vi "Write Configuration.vi"(8 "error in (no error)":errorcluster, 10 "Configuration.lvlibp:Configuration.lvclass":refnum<class "Configuration.lvclass">, 11 "BFECC in":refnum<class "BFECC.lvclass">) -> (0 "error out":errorcluster, 3 "BFECC out":refnum<class "BFECC.lvclass">)   [LabVIEW 2018, in "BFECC.lvlib" / "BFECC.lvclass"]
uses:
  BFECC.lvclass
  AME Test Engineering/LabVIEW/PPLs/Configuration/Configuration.lvlibp/Configuration.lvclass
  BFECC.lvclass/BFECC.ctl
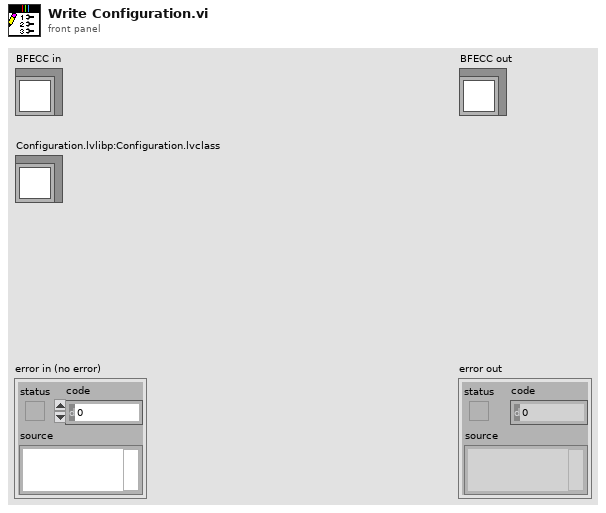
[diagram p1: front panel]
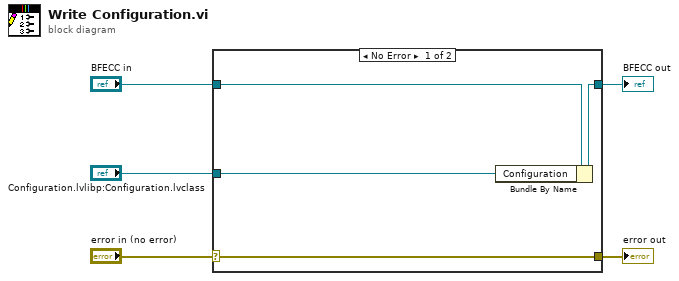
[diagram p0: block diagram]
diagram:
  n1 = case shown="No Error" "error in (no error)" {
    selector: "error in (no error)" -> [w9 w10]
    tunnel: [w9 w10] -> w4
    tunnel: [w7 w11] -> w2
    tunnel: "BFECC in" -> [w8 w11]
    tunnel: "Configuration.lvlibp:Configuration.lvclass" -> [w6 _]
    frame No Error {
      n2 = Bundle By Name(cluster=w8, "Configuration"=w6) -> (w7:refnum<class "BFECC.lvclass">)
    }
    frame Error {
    }
  }
  "error out" <- w4
  "BFECC out" <- w2
